vi "Measure current and save data.vi"(5 "Voltage1":dbl, 7 "Voltage 0":dbl, 8 "error in (no error)":errorcluster, 9 "Barcode2":string, 10 "Barcode1":string, 11 "BoardHandle in 5":T1) -> (0 "error out":errorcluster, 3 "BoardHandle out 3":T1)   [LabVIEW 2020]
uses:
  <instrlib>/CAEN PSM/CAEN PSM.lvlib
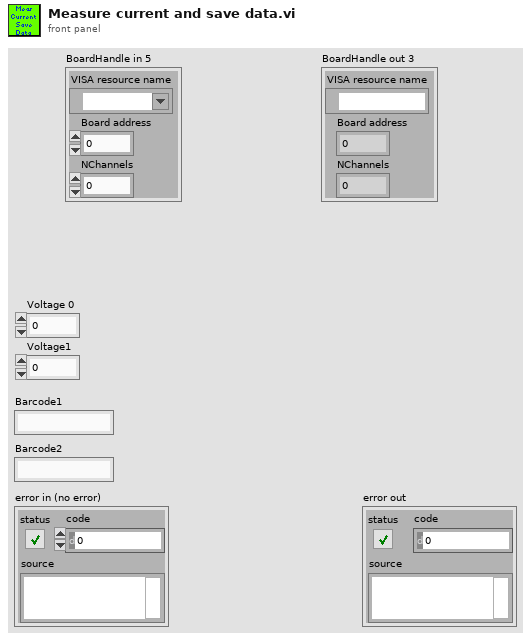
[diagram p1: front panel]
types:
  T1 = cluster{"VISA resource name":refnum<visa-resource-name>, "Board address":u8, "NChannels":u8}
  T2 = typedef "CAEN PSM.lvlib/BoardHandle.ctl" = cluster{"VISA resource name":refnum<visa-resource-name>, "Board address":i8, "NChannels":u8}
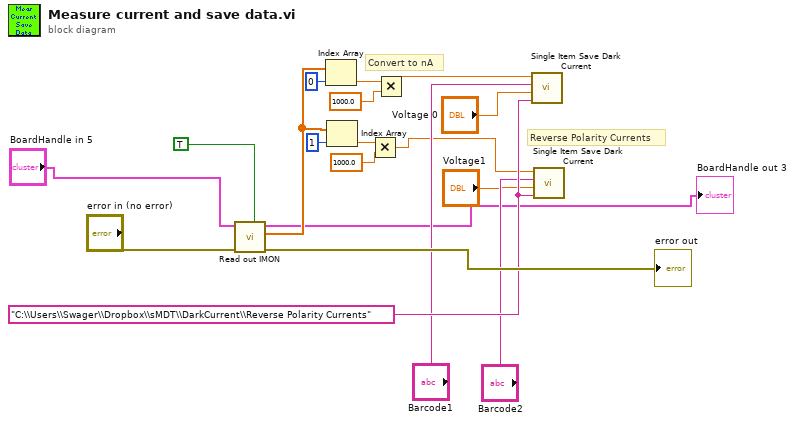
[diagram p0: block diagram]
diagram:
  w18 = "C:\\Users\\Swager\\Dropbox\\sMDT\\DarkCurrent\\Reverse Polarity Currents" ("Filename")
  # "Reverse Polarity Currents"
  # "Convert to nA"
  n1 = call <instrlib>:"Read out IMON.vi"("All Channels (T)"=TRUE ("All Channels (F)"), "error in (no error)"="error in (no error)", "BoardHandle"="BoardHandle in 5") -> ("error out"=→"error out":errorcluster, "IMon values (uA)"=w13:dbl[], "BoardHandle out"=→"BoardHandle out 3":T2)  [unwired: 5 in, 1 out]
  n2 = Index Array(array=w13, index=0) -> (element=w10:dbl)
  n3 = Index Array(array=w13, index=1) -> (element=w7:dbl)
  n4 = Multiply(x=w7, y=1000.0) -> (x*y=w15:dbl)
  n5 = Multiply(x=w10, y=1000.0) -> (x*y=w14:dbl)
  n6 = call "Single Item Save Dark Current.vi"("Filename"=w18, "Voltage"="Voltage 0", "Barcode"="Barcode1", "Current"=w14) -> ()  [unwired: 8 in]
  n7 = call "Single Item Save Dark Current.vi"("Filename"=w18, "Voltage"="Voltage1", "Barcode"="Barcode2", "Current"=w15) -> ()  [unwired: 8 in]
